vi "fgv_stop_agv.vi"(7 "cmd":enum16{"ini", "read", "stop"}(ring)) -> (3 "stop status":bool)   [LabVIEW 2019]
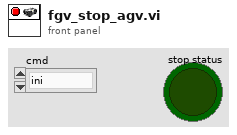
[diagram p1: front panel]
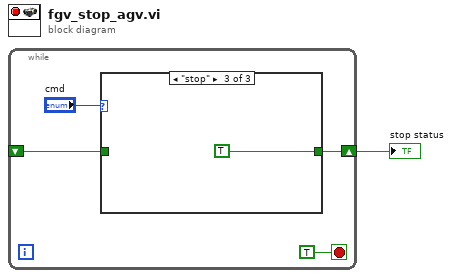
[diagram p0: block diagram]
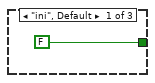
[diagram p2: hidden frame]
diagram:
  n1 = while {
    shift-right: [w3] -> w1
    shift-left: _ -> [w2]
    stop <- TRUE stop-if-true
    n2 = case shown="\"stop\"" "cmd" {
      tunnel: [FALSE w7 TRUE] -> w3
      tunnel: w2 -> [_ w7 _]
      frame "ini", Default {
      }
      frame "read" {
      }
      frame "stop" {
      }
    }
  }
  "stop status" <- w1
